vi "ASI Set Start Pos.vi"(9 "iStartY":i32, 10 "iStartX":i32, 11 "iCameraID":i32) -> (3 "function return":i32)   [LabVIEW 2023, in "ASICamera2_no_err.lvlib"]
doc: "ASICAMERA_API ASI_ERROR_CODE ASISetStartPos(int iCameraID, int iStartX, int iStartY);"
uses:
  ASICamera2_no_err.lvlib
  LabviewDAQ-master/ConcreteClasses/ConcreteInstrumentClasses/CameraClasses/ZWO_ASI_LV/Labview_ASI_demo_64bit_221128/user.lib/ASICamera2_no_err/ASICamera2.dll
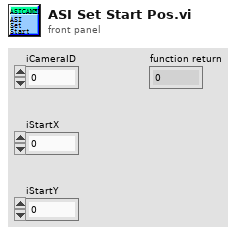
[diagram p1: front panel]
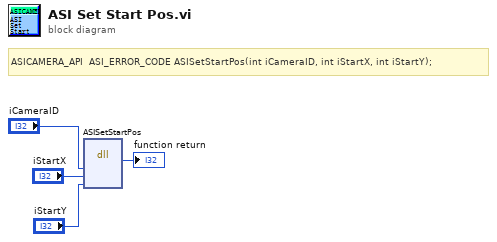
[diagram p0: block diagram]
diagram:
  # "ASICAMERA_API  ASI_ERROR_CODE ASISetStartPos(int iCameraID, int iStartX, int iStartY);"
  n1 = dll-call lib="W:/Quant_Opt_Group/Group/Alex/LabviewDAQ-master/ConcreteClasses/ConcreteInstrumentClasses/CameraClasses/ZWO_ASI_LV/Labview_ASI_demo_64bit_221128/user.lib/ASICamera2_no_err/ASICamera2.*" fn="ASISetStartPos"("iCameraID"="iCameraID", "iStartX"="iStartX", "iStartY"="iStartY") -> (→"function return":i32)  [unwired: 6 in, 2 out]
